vi "linear_x.vi"(0 "Byte Stream File in":refnum<file>, 2 "Array":dbl[](array[numeric]), 5 "base path":path, 7 "Record  SS 661":bool, 9 "Boolean 3":bool, 11 "error in (no error)":errorcluster, 12 "Initial Time in":timestamp, 13 "Stop Program 4":bool) -> (4 "Byte Stream File out":refnum<file>, 6 "Boolean 2":bool, 8 "Initial Time out":timestamp, 10 "Stop Program 5":bool, 15 "error out":errorcluster)   [LabVIEW 2014]
uses:
  Program Files (x86)/National Instruments/LabVIEW 2014/vi.lib/addons/database/Connection.llb/DB Tools Open Connec (String).vi
  Program Files (x86)/National Instruments/LabVIEW 2014/vi.lib/addons/database/Connection.llb/Conn Execute.vi
  Program Files (x86)/National Instruments/LabVIEW 2014/vi.lib/addons/database/Recordset.llb/Rec Destroy - Connection.vi
  Program Files (x86)/National Instruments/LabVIEW 2014/vi.lib/addons/database/NI_Database_API.lvlib
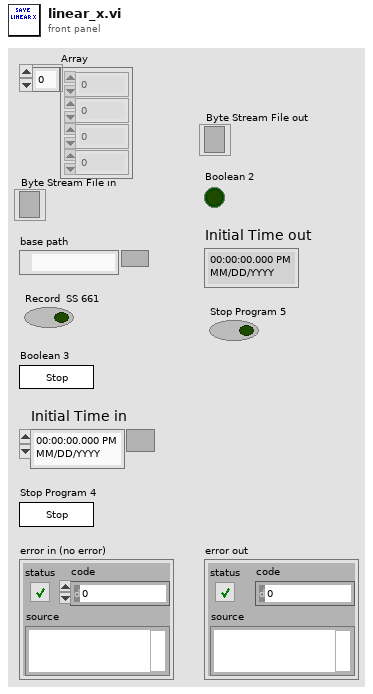
[diagram p1: front panel]
types:
  T1 = cluster{"Array":dbl[], "seconds since 1Jan1904":timestamp}
  T2 = enum16{"NotSaving", "Create", "Reading", "Closing"}
  T3 = typedef "NI_Database_API.lvlib/Conn ObjectReference.ctl" = refnum<k1>
  T4 = enum16{"open", "replace", "create", "open or create", "replace or create", "replace or create with confirmation"}
  T5 = typedef "NI_Database_API.lvlib/Rec ObjectReference.ctl" = refnum<k1>
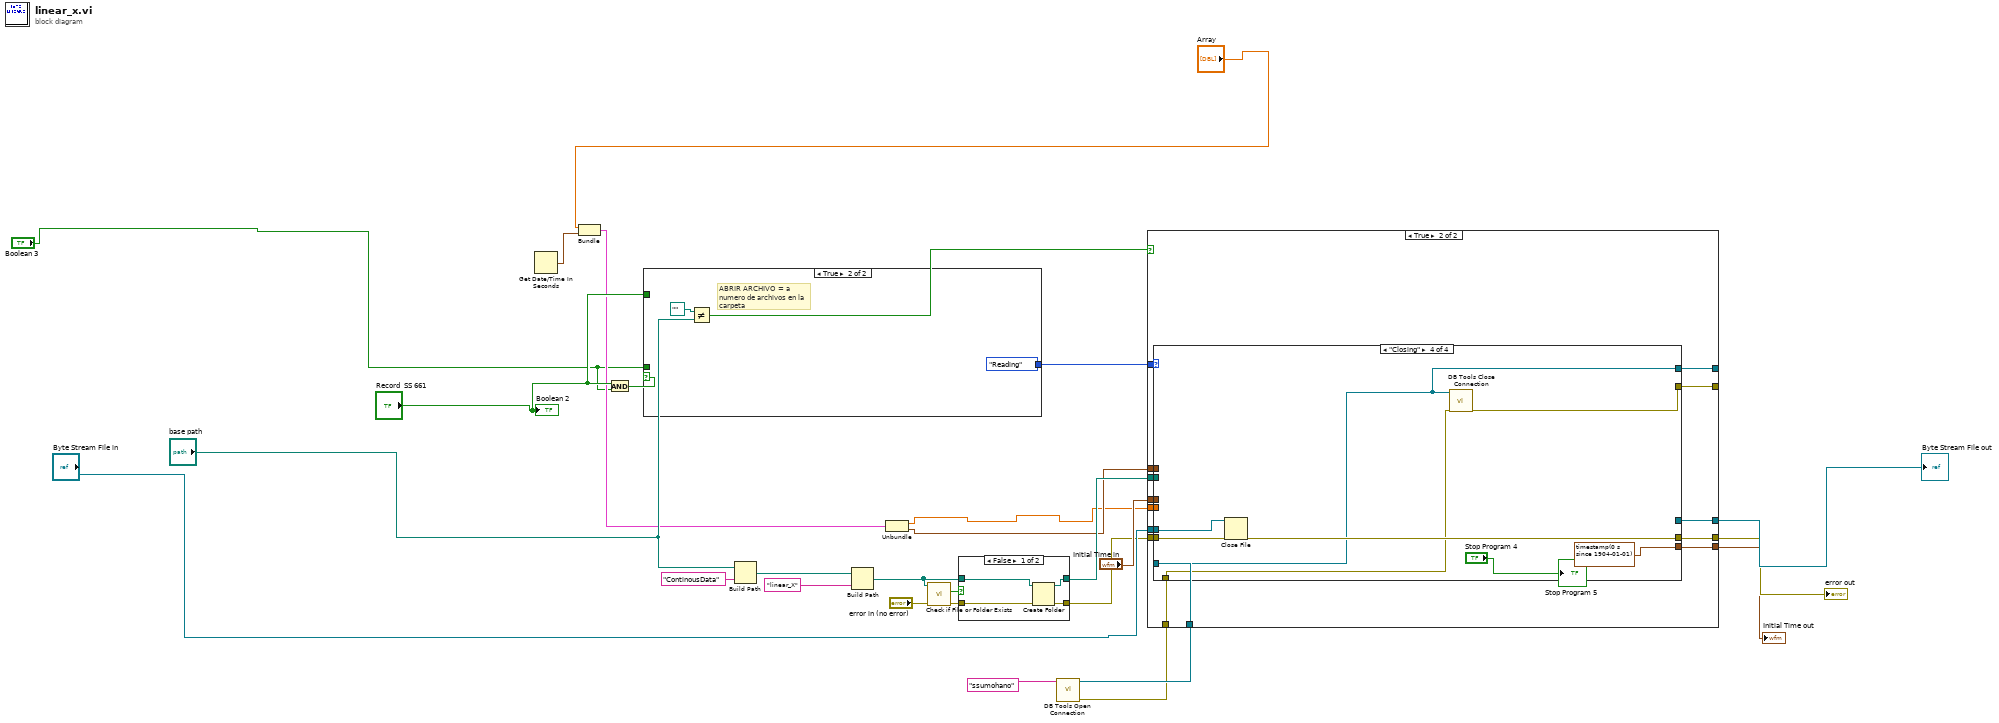
[diagram p0: block diagram]
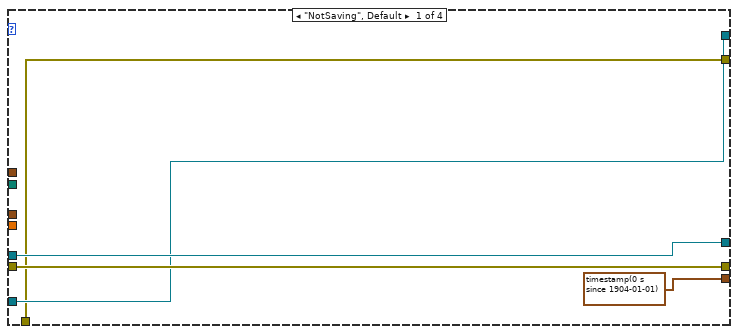
[diagram p4: hidden frame]
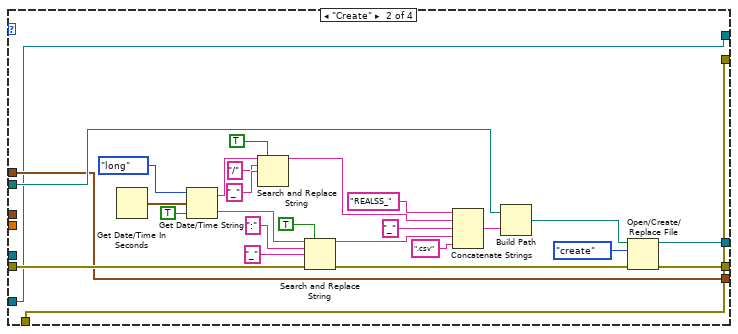
[diagram p5: hidden frame]
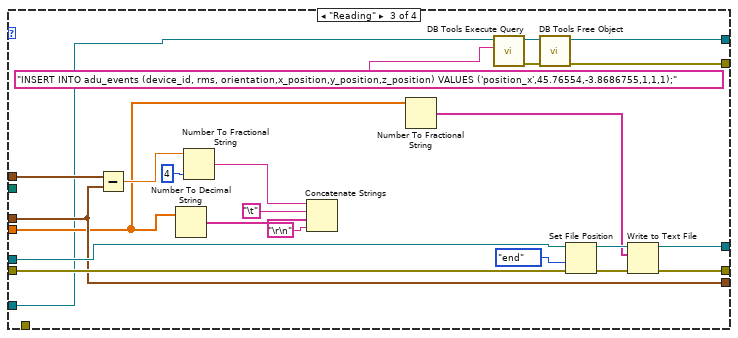
[diagram p6: hidden frame]
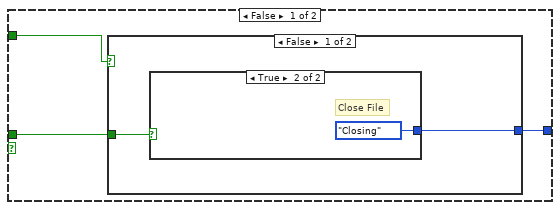
[diagram p7: hidden frame]
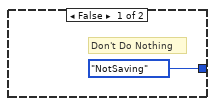
[diagram p8: hidden frame]
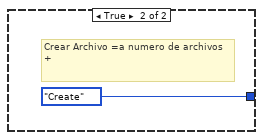
[diagram p9: hidden frame]
diagram:
  n1 = Get Date/Time In Seconds() -> (seconds since 1Jan1904=w9:timestamp)
  n2 = Bundle("Array"="Array", "seconds since 1Jan1904"=w9) -> (w8:T1)  [unwired: 1 in]
  n3 = And(x="Record  SS 661", y="Boolean 3") -> (x .and. y?=w24:bool)
  n4 = case shown="True" w24 {
    tunnel: "Boolean 3" -> [w33 _]
    tunnel: [w32 T2."Reading" ("Enum")] -> w23
    tunnel: "Record  SS 661" -> [w31 _]
    frame False {
      n5 = case shown="False" w31 {
        tunnel: w33 -> [w35 _]
        tunnel: [w34 T2."Create" ("Enum")] -> w32
        frame False {
          n6 = case shown="True" w35 {
            tunnel: [T2."NotSaving" ("Enum") T2."Closing" ("Enum")] -> w34
            frame False {
              # "Don't Do Nothing"
            }
            frame True {
              # "Close File"
            }
          }
        }
        frame True {
          # "Crear Archivo =a numero de archivos +"
        }
      }
    }
    frame True {
      # "ABRIR ARCHIVO = a numero de archivos en la carpeta"
    }
  }
  n7 = Not Equal?(x=path "" ("Project Folder"), y="base path") -> (x != y?=w17:bool)
  n8 = Build Path(base path="base path", name or relative path="ContinousData") -> (appended path=w13:path)
  n9 = Build Path(base path=w13, name or relative path="linear_X") -> (appended path=w12:path)
  n10 = Unbundle(w8) -> ("Array"=w6:dbl[], "seconds since 1Jan1904"=w7:timestamp)
  n11 = call <vilib>:"Check if File or Folder Exists.vi"("error in (no error)"="error in (no error)", "path"=w12) -> ("error out"=w15:errorcluster, "file or folder exists?"=w16:bool)  [unwired: 7 in, 1 out]
  n12 = case shown="False" w16 {
    tunnel: [w43 w45] -> w10
    tunnel: w15 -> [w42 w45]
    tunnel: w12 -> [w41 w44]
    tunnel: [w40 w44] -> w11
    frame False {
      n13 = Create Folder(path (use dialog)=w41, error in=w42) -> (created path=w40:path, error out=w43:errorcluster)  [unwired: 1 in, 1 out]
    }
    frame True {
    }
  }
  n14 = call-poly "DB Tools Open Connection.vi"("connection information"="ssumohano") -> ("error out"=w1:errorcluster, "connection reference"=w2:T3)  [unwired: 7 in]
  n15 = case shown="True" w17 {
    tunnel: w11 -> [_ w60]
    tunnel: w6 -> [_ w62]
    tunnel: w23 -> [_ w61]
    tunnel: w10 -> [w48 w59]
    tunnel: "Byte Stream File in" -> [_ w58]
    tunnel: [_ w57] -> w29
    tunnel: [w48 w56] -> w22
    tunnel: [_ w55] -> w21
    tunnel: "Initial Time in" -> [_ w54]
    tunnel: w7 -> [_ w53]
    tunnel: w2 -> [w46 w52]
    tunnel: [w47 w51] -> _
    tunnel: [w46 w49] -> _
    tunnel: w1 -> [w47 w50]
    frame False {
    }
    frame True {
      n16 = case shown="\"Closing\"" w61 {
        tunnel: w62 -> [_ _ w102 _]
        tunnel: w60 -> [_ w94 _ _]
        tunnel: w59 -> [w67 w75 w113 w124]
        tunnel: w58 -> [w66 _ w116 w122]
        tunnel: [w66 w73 w109 _] -> w57
        tunnel: [w67 w72 w110 w123] -> w56
        tunnel: [timestamp(0 s since 1904-01-01) ("Initial Time") w70 w108 timestamp(0 s since 1904-01-01) ("Initial Time")] -> w55
        tunnel: w54 -> [_ _ w108 _]
        tunnel: w53 -> [_ w70 w107 _]
        tunnel: w52 -> [w64 w69 w97 w119]
        tunnel: [w64 w69 w96 w119] -> w49
        tunnel: [w63 w68 w95 w118] -> w51
        tunnel: w50 -> [w63 w68 _ w120]
        frame "NotSaving", Default {
        }
        frame "Create" {
          n17 = Get Date/Time In Seconds() -> (seconds since 1Jan1904=w91:timestamp)
          n18 = Get Date/Time String(date format (0)=enum16{"short", "long", "abbreviated"}."long", seconds (now)=w91, want seconds? (F)=TRUE) -> (date string=w89:string, time string=w85:string)
          n19 = Search and Replace String(replace all?=TRUE ("replace all? (F)"), input string=w89, search string="/", replace string="_" ("replace string (\"\")")) -> (result string=w82:string)  [unwired: 4 in, 3 out]
          n20 = Search and Replace String(replace all?=TRUE ("replace all? (F)"), input string=w85, search string=":", replace string="_" ("replace string (\"\")"), error in=w75) -> (result string=w80:string, error out=w76:errorcluster)  [unwired: 3 in, 2 out]
          n21 = Concatenate Strings("REALSS_" ("string"), w82, "_" ("string"), w80, ".csv" ("string")) -> (w78:string)
          n22 = Build Path(base path=w94, name or relative path=w78) -> (appended path=w93:path)
          n23 = Open/Create/Replace File(file path (use dialog)=w93, error in=w76, operation (0:open)=T4."create") -> (refnum out=w73:refnum<file>, error out=w72:errorcluster)  [unwired: 3 in, 1 out]
        }
        frame "Reading" {
          n24 = Subtract(x=w107, y=w108) -> (x-y=w105:dbl)
          n25 = Number To Decimal String(number=w102) -> (decimal integer string=w112:string[])  [unwired: 1 in]
          n26 = Number To Fractional String(number=w105, precision (6)=i16 4) -> (F-format string=w103:string)  [unwired: 2 in]
          n27 = Concatenate Strings(w103, "\t", w112, "\r\n") -> ()  [unwired: 1 out]
          n28 = Number To Fractional String(number=w102) -> (F-format string=w101:string[])  [unwired: 3 in]
          n29 = call-poly "DB Tools Execute Query.vi"("SQL query"="INSERT INTO adu_events (device_id, rms, orientation,x_position,y_position,z_position) VALUES ('position_x',45.76554,-3.8686755,1,1,1);", "connection reference"=w97) -> ("error out"=w100:errorcluster, "recordset reference"=w99:T5)  [unwired: 6 in]
          n30 = call-poly "DB Tools Free Object.vi"("error in (no error)"=w100, "recordset reference"=w99) -> ("error out"=w95:errorcluster, "connection reference"=w96:T3)  [unwired: 8 in]
          n31 = Set File Position(refnum=w116, from (0:start)=enum16{"start", "end", "current"}."end", error in=w113) -> (refnum out=w115:refnum<file>, error out=w114:errorcluster)  [unwired: 1 in]
          n32 = Write to Text File(file (use dialog)=w115, text=w101, error in=w114) -> (refnum out=w109:refnum<file>, error out=w110:errorcluster)  [unwired: 1 in, 1 out]
        }
        frame "Closing" {
          n33 = Close File(refnum=w122, error in=w124) -> (error out=w123:errorcluster)  [unwired: 1 out]
          n34 = call "DB Tools Close Connection.vi"("error in (no error)"=w120, "connection reference"=w119) -> ("error out"=w118:errorcluster)  [unwired: 5 in]
        }
      }
    }
  }
  "error out" <- w22
  "Initial Time out" <- w21
  "Byte Stream File out" <- w29
  "Boolean 2" <- "Record  SS 661"
  "Stop Program 5" <- "Stop Program 4"
